vi "Post Substeps Waveform Generation Task Stop.vi"(10 "Socket No":u16=1, 11 "Sequence Context In":refnum<k7>) -> (0 "error out":errorcluster, 3 "Report Text":string)   [LabVIEW 2023, in "LTT_TeststandSteptypes.lvlib"]
doc: "This VI Is Socket Number based AO Data Signal Write Through Q"
uses:
  LTT_TeststandSteptypes.lvlib
panel:
  in  "AOWrite":T1 {"Signal Name List"."Waveform Type" items=["Sine Wave", "Triangle Wave", "Square Wave", "Sawtooth Wave"]}
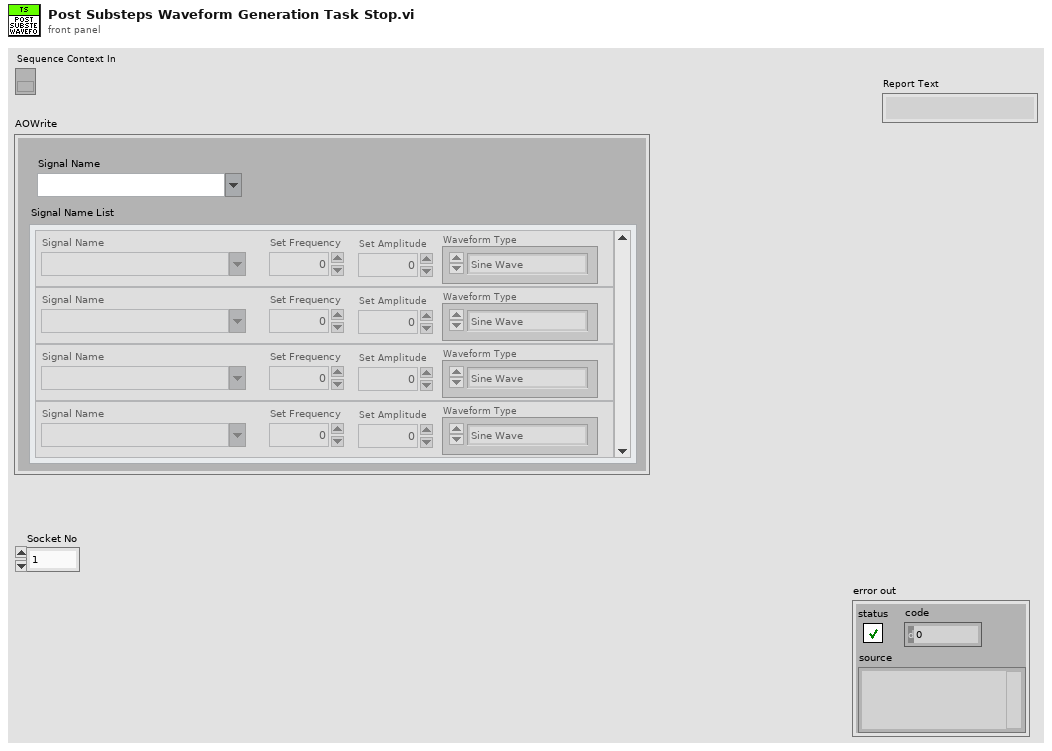
[diagram p1: front panel]
types:
  T1 = cluster{"Signal Name":string, "Signal Name List":cluster{"Signal Name":string, "Set Frequency":dbl, "Set Amplitude":dbl, "Waveform Type":u16}[]}
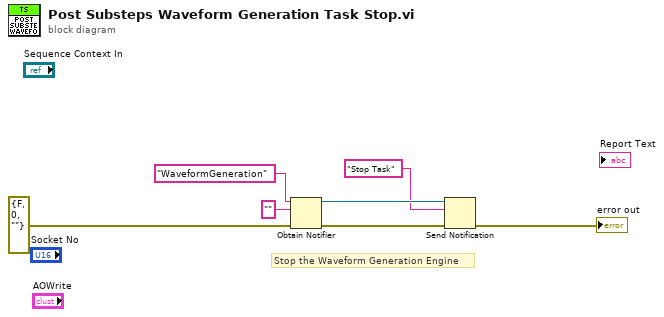
[diagram p0: block diagram]
diagram:
  # "Stop the Waveform Generation Engine"
  n1 = Obtain Notifier(name (unnamed)="WaveformGeneration", notification data type="", error in (no error)=errorcluster {"status"=FALSE, "code"=0, "source"=""} ("error in")) -> (notifier out=w3:refnum<notifier>, error out=w4:errorcluster)  [unwired: 1 in, 1 out]
  n2 = Send Notification(notification="Stop Task", notifier=w3, error in (no error)=w4) -> (error out=→"error out":errorcluster)  [unwired: 1 out]
